vi "WFS Convert Wavefront Waves.vi"(8 "error in (no error)":errorcluster {"code" format="%.0x"}, 9 "Array Wavefront In":u32, 10 "Wavelength":dbl, 11 "instrument handle":refnum<visa-resource-name>) -> (0 "error out":errorcluster {"code" format="%.0x"}, 2 "Array Wavefront Out":u32, 3 "instrument handle out":refnum<visa-resource-name>)   [LabVIEW 2020]
doc: "This VI converts the wavefront data array calculated by VI CalcWavefront() from µm into waves unit depending on the actual wavelength."
uses:
  WFS_32.dll
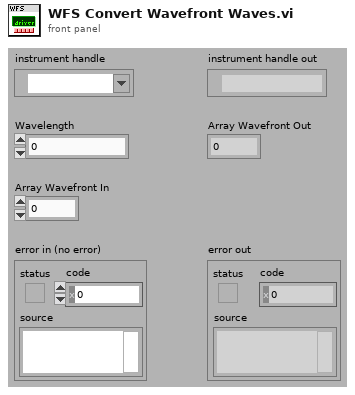
[diagram p1: front panel]
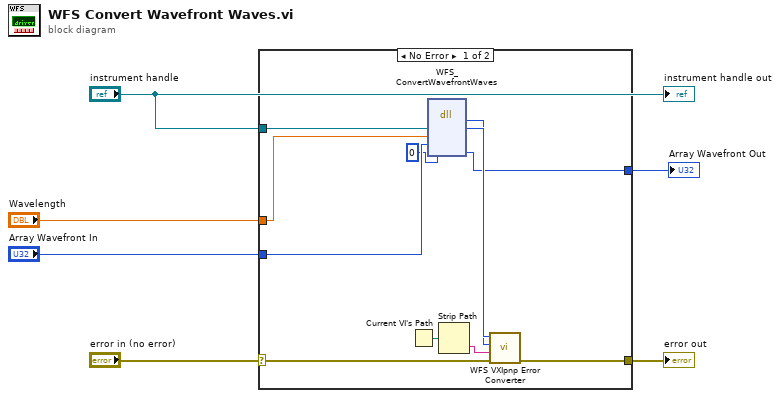
[diagram p0: block diagram]
diagram:
  n1 = case shown="No Error" "error in (no error)" {
    selector: "error in (no error)" -> [w12 w18]
    tunnel: [w11 w18] -> w6
    tunnel: "instrument handle" -> [w16 _]
    tunnel: "Wavelength" -> [w10 _]
    tunnel: "Array Wavefront In" -> [w9 _]
    tunnel: [w7 _] -> w1
    frame No Error {
      n2 = Current VI's Path() -> (path=w17:path)
      n3 = dll-call lib="WFS_*.*" fn="WFS_ConvertWavefrontWaves"("Instrument Handle"=w16, "Wavelength"=w10, "Array Wavefront In"=w9, "Array Wavefront Out"=u32 0) -> (w14:i32, "Instrument Handle"=w15:u32, "Array Wavefront Out"=w7:u32)  [unwired: 5 in, 2 out]
      n4 = Strip Path(path=w17) -> (name=w13:string)  [unwired: 1 out]
      n5 = call "WFS VXIpnp Error Converter.vi"("error in (no error)"=w12, "Name Of VI (\"\")"=w13, "CVI Error Code (0)"=w14, "instrument handle"=w15) -> ("error out"=w11:errorcluster)  [unwired: 6 in, 1 out]
    }
    frame Error {
    }
  }
  "error out" <- w6
  "Array Wavefront Out" <- w1
  "instrument handle out" <- "instrument handle"
